vi "G#Object_Create.vi"(0 "reference in":refnum<class "G#SubSubClass1.lvclass">, 3 "control values":variant[](array[variant]), 5 "error in (no error)":errorcluster) -> (14 "reference out":refnum<class "G#SubSubClass1.lvclass">, 19 "error out":errorcluster)   [LabVIEW 2010, in "G#SubSubClass1.lvclass"]
uses:
  G#SubSubClass1.lvclass
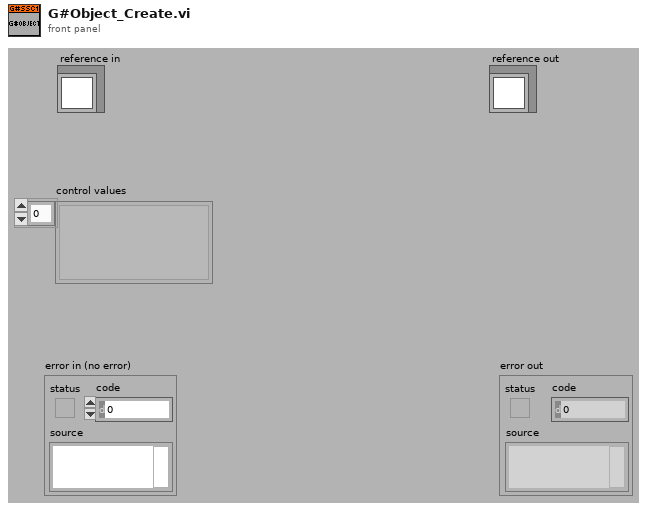
[diagram p1: front panel]
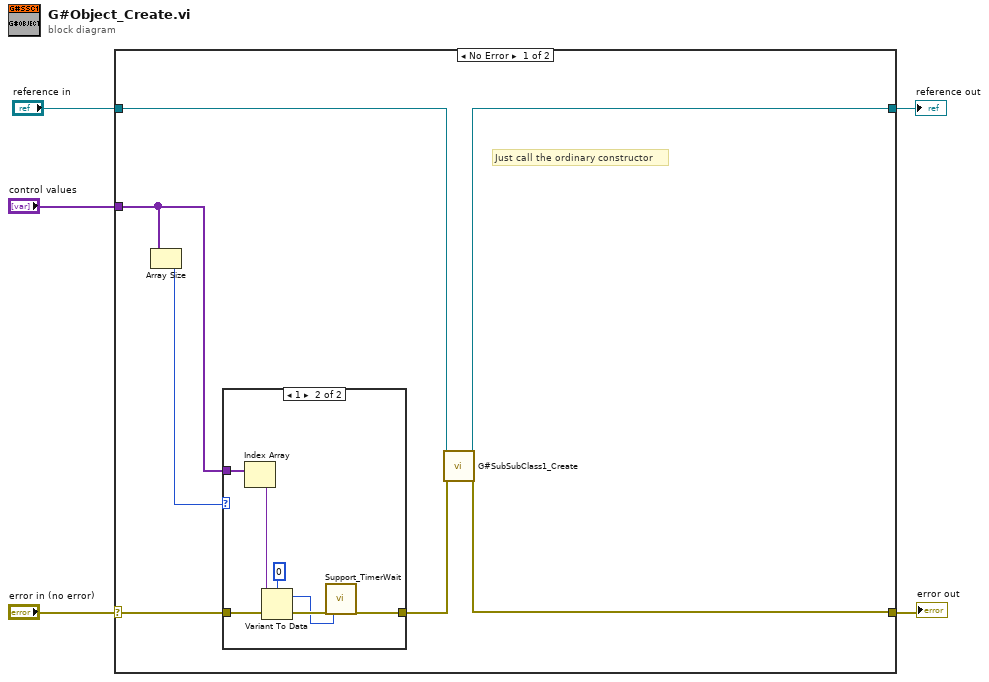
[diagram p0: block diagram]
diagram:
  n1 = case shown="No Error" "error in (no error)" {
    selector: "error in (no error)" -> [w9 w22]
    tunnel: [w12 w22] -> w4
    tunnel: [w10 w21] -> w2
    tunnel: "reference in" -> [w11 w21]
    tunnel: "control values" -> [w6 _]
    frame No Error {
      # "Just call the ordinary constructor"
      n2 = Array Size(array=w6) -> (size(s)=w7:i32)
      n3 = case shown="1" w7 {
        tunnel: w9 -> [w13 w20]
        tunnel: [w13 w17] -> w8
        tunnel: w6 -> [_ w18]
        frame 0, Default {
        }
        frame 1 {
          n4 = Index Array(array=w18) -> (element=w19:variant)  [unwired: 1 in]
          n5 = Variant To Data(error in=w20, Variant=w19, type=u32 0 ("milliseconds to wait")) -> (error out=w16:errorcluster, data=w14:u32)
          n6 = call "Support_TimerWait.vi"("error in (no error)"=w16, "milliseconds to wait"=w14) -> ("error out"=w17:errorcluster)  [unwired: 17 in]
        }
      }
      n7 = call "G#SubSubClass1_Create.vi"("reference in"=w11, "error in (no error)"=w8) -> ("reference out"=w10:refnum<class "G#SubSubClass1.lvclass">, "error out"=w12:errorcluster)  [unwired: 16 in]
    }
    frame Error {
    }
  }
  "error out" <- w4
  "reference out" <- w2
